vi "52-lfs-r1.vi"(8 "error in (no error)":errorcluster, 9 "Position in":T1) -> (0 "error out":errorcluster, 1 "Position out":T1)   [LabVIEW 2019]
uses:
  subVI/move/position cluster.ctl
  subVI/move control/move and align/move_cluster.ctl
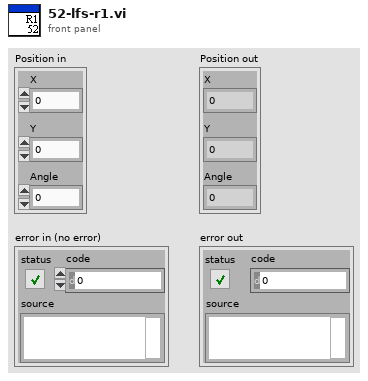
[diagram p1: front panel]
types:
  T1 = typedef "position cluster.ctl" = cluster{"X":dbl, "Y":dbl, "Angle":dbl}
  T2 = typedef "move_cluster.ctl" = cluster{"X":dbl, "Y":dbl, "degree":dbl, "speed":dbl}
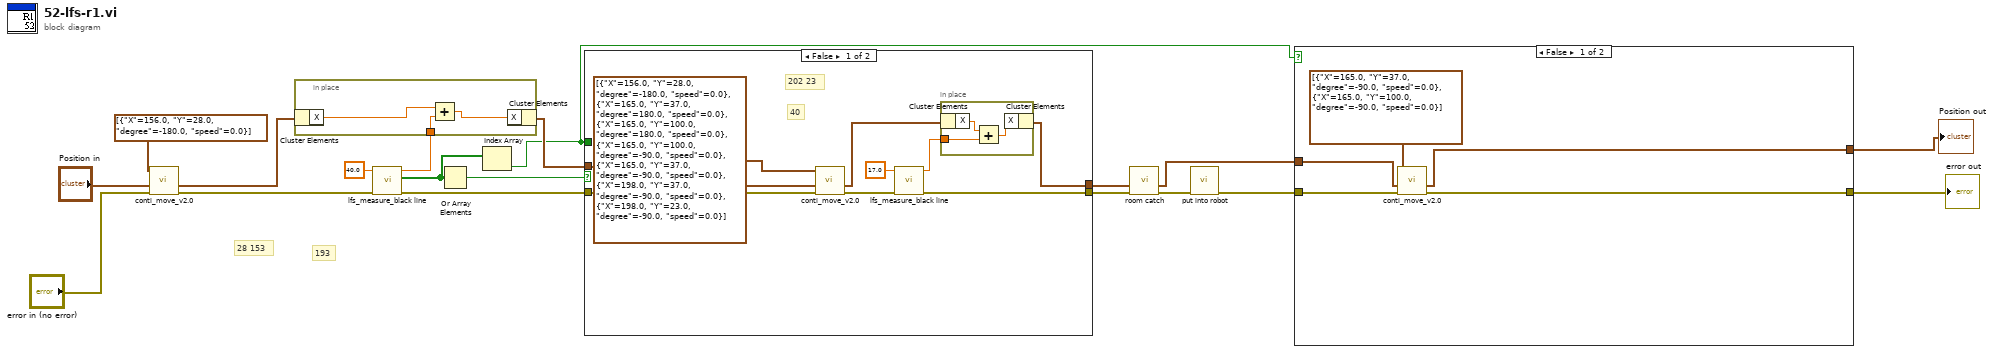
[diagram p0: block diagram]
diagram:
  # "193"
  # "28 153"
  n1 = call "conti_move_v2.0.vi"("error in (no error)"="error in (no error)", "Position"="Position in", "route"=T2[] [{"X"=156.0, "Y"=28.0, "degree"=-180.0, "speed"=0.0}]) -> ("error out"=w19:errorcluster, "Position out"=w14:T1)  [unwired: 7 in]
  n2 = call "lfs_measure_black line.vi"("error in (no error)"=w19, "limit"=40.0) -> ("error out"=w11:errorcluster, "0:R 1:L"=w9:bool[], "move cm"=w13:dbl)  [unwired: 7 in]
  n3 = in-place {
    in-place-border: w13 -> [w21]
    n4 = in-place-cluster #1(w14) -> ("X"=w22:dbl)
    n5 = Add(x=w22, y=w21) -> (x+y=w20:dbl)
    n6 = in-place-cluster #1("X"=w20) -> (w10:T1)
  }
  n7 = Or Array Elements(Boolean array=w9) -> (logical OR=w12:bool)
  n8 = Index Array(array=w9) -> (element=w5:bool)  [unwired: 1 in]
  n9 = case shown="False" w12 {
    tunnel: w11 -> [w31 w36]
    tunnel: w10 -> [w30 w35]
    tunnel: w5 -> [_ _]
    tunnel: [w24 w36] -> w7
    tunnel: [w23 w35] -> w6
    frame False {
      # "40"
      # "202 23"
      n10 = call "conti_move_v2.0.vi"("error in (no error)"=w31, "Position"=w30, "route"=T2[] [{"X"=156.0, "Y"=28.0, "degree"=-180.0, "speed"=0.0}, {"X"=165.0, "Y"=37.0, "degree"=180.0, "speed"=0.0}, {"X"=165.0, "Y"=100.0, "degree"=180.0, "speed"=0.0}, {"X"=165.0, "Y"=100.0, "degree"=-90.0, "speed"=0.0}, {"X"=165.0, "Y"=37.0, "degree"=-90.0, "speed"=0.0}, {"X"=198.0, "Y"=37.0, "degree"=-90.0, "speed"=0.0}, {"X"=198.0, "Y"=23.0, "degree"=-90.0, "speed"=0.0}]) -> ("error out"=w28:errorcluster, "Position out"=w26:T1)  [unwired: 7 in]
      n11 = call "lfs_measure_black line.vi"("error in (no error)"=w28, "limit"=17.0) -> ("error out"=w24:errorcluster, "move cm"=w25:dbl)  [unwired: 7 in, 1 out]
      n12 = in-place {
        in-place-border: w25 -> [w33]
        n13 = in-place-cluster #2(w26) -> ("X"=w34:dbl)
        n14 = Add(x=w34, y=w33) -> (x+y=w32:dbl)
        n15 = in-place-cluster #2("X"=w32) -> (w23:T1)
      }
    }
    frame True {
    }
  }
  n16 = call "room catch.vi"("error in (no error)"=w7, "Position in"=w6) -> ("error out"=w8:errorcluster, "Position out 2"=w3:T1)  [unwired: 8 in]
  n17 = call "put into robot.vi"("error in (no error)"=w8) -> ("error out"=w4:errorcluster)  [unwired: 10 in]
  n18 = case shown="False" w5 {
    tunnel: w4 -> [w41 w43]
    tunnel: w3 -> [w39 w42]
    tunnel: [w38 w43] -> w2
    tunnel: [w37 w42] -> w1
    frame False {
      n19 = call "conti_move_v2.0.vi"("error in (no error)"=w41, "Position"=w39, "route"=T2[] [{"X"=165.0, "Y"=37.0, "degree"=-90.0, "speed"=0.0}, {"X"=165.0, "Y"=100.0, "degree"=-90.0, "speed"=0.0}]) -> ("error out"=w38:errorcluster, "Position out"=w37:T1)  [unwired: 7 in]
    }
    frame True {
    }
  }
  "Position out" <- w1
  "error out" <- w2
